vi "Create Axis.vi"(7 "Axis label?":bool, 8 "error in (no error)":errorcluster, 9 "Half plane?":bool, 10 "Show Axis":bool, 11 "SceneObject in":refnum<vi>) -> (0 "error out":errorcluster, 3 "SceneObject out":refnum<vi>)   [LabVIEW 2013]
doc: "This VI adds an axis with length 2, radius 0.03 to a SceneObject."
uses:
  <vilib>/picture/3D Picture Control/Object/Add Object (no reference).vi
  <vilib>/picture/3D Picture Control/NI_3D Picture Control.lvlib
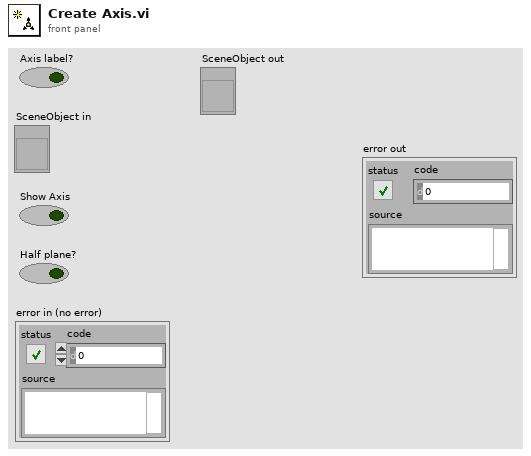
[diagram p1: front panel]
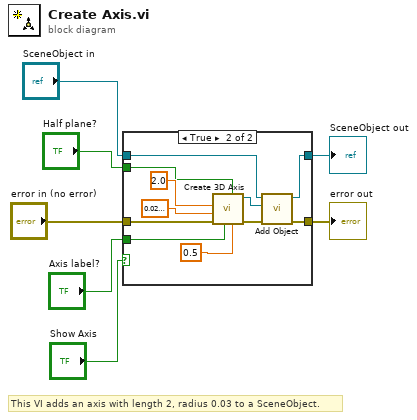
[diagram p0: block diagram]
diagram:
  # "This VI adds an axis with length 2, radius 0.03 to a SceneObject."
  n1 = case shown="True" "Show Axis" {
    tunnel: [w9 w13] -> w7
    tunnel: "Half plane?" -> [_ w18]
    tunnel: [w8 w10] -> w1
    tunnel: "Axis label?" -> [_ w17]
    tunnel: "SceneObject in" -> [w9 w15]
    tunnel: "error in (no error)" -> [w8 w12]
    frame False {
      # "Pass an empty model when displaying no axis."
    }
    frame True {
      # "Add a 3D axis."
      n2 = call <vilib>:"Create 3D Axis.vi"("Character Size"=sgl 0.5, "Half plane?"=w18, "Axis label?"=w17, "error in (no error)"=w12, "Radius"=sgl 0.03, "Length"=sgl 2.0 ("Height")) -> ("error out"=w11:errorcluster, "New Object Refnum"=w14:refnum<vi>)  [unwired: 4 in]
      n3 = call-poly <vilib>:"Add Object.vi"("error in (no error)"=w11, "New Object In"=w14, "Scene Object In"=w15) -> ("error out"=w10:errorcluster, "Scene Object Out"=w13:refnum<vi>)  [unwired: 7 in]
    }
  }
  "SceneObject out" <- w7
  "error out" <- w1
